vi "Get class reference.vi"() -> (0 "BaseClass.lvclass":refnum<class "BaseClass.lvclass">)   [LabVIEW 2022 SP3, in "BaseClass.lvclass"]
uses:
  BaseClass.lvclass
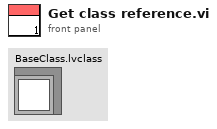
[diagram p1: front panel]
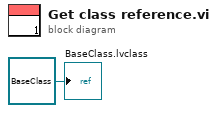
[diagram p0: block diagram]
diagram:
  "BaseClass.lvclass" <- refnum<class "BaseClass.lvclass"> refnum ("BaseClass.lvclass")
